vi "Write OVP_Enable.vi"(8 "error in":errorcluster, 10 "OVP_Enable":bool, 11 "36234A in":refnum<class "36234A.lvclass">) -> (0 "error out":errorcluster, 3 "36234A out":refnum<class "36234A.lvclass">)   [LabVIEW 2019, in "36234A.lvlib" / "36234A.lvclass"]
uses:
  Library/36234A.lvclass
  C:/Users/Public/Documents/Development/builds/Instruments/PowerSupply.lvlibp/Library/PowerSupply.lvclass
  builds/Instruments/PowerSupply.lvlibp/Accessors/Read Active Channel.vi
  builds/Instruments/PowerSupply.lvlibp/Library/PowerSupply.lvclass
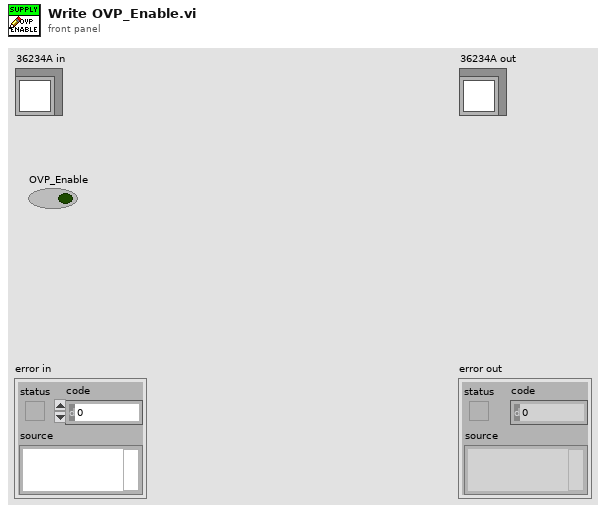
[diagram p1: front panel]
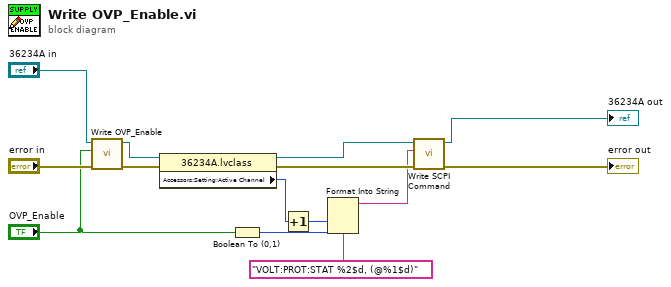
[diagram p0: block diagram]
diagram:
  n1 = call-parent "Write OVP_Enable.vi"("error in"="error in", "OVP_Enable"="OVP_Enable", "PowerSupply in"="36234A in") -> ("error out"=w14:errorcluster, "PowerSupply out"=w11:refnum<class "36234A.lvclass">)  [unwired: 7 in]
  n2 = property class="36234A.lvclass"(reference=w11, error in=w14) -> (reference out=w6:refnum<class "36234A.lvclass">, error out=w5:errorcluster, "Accessors:Setting:Active Channel"=w7:u32)
  n3 = Boolean To (0,1)(Boolean="OVP_Enable") -> (0, 1=w8:i16)
  n4 = Increment(x=w7) -> (x+1=w1:u32)
  n5 = Format Into String(format string="VOLT:PROT:STAT %2$d, (@%1$d)", w1, w8) -> (resulting string=w2:string)  [unwired: 2 in, 1 out]
  n6 = call "Write SCPI Command.vi"("error in (no error)"=w5, "SCPI Command"=w2, "36234A in"=w6) -> ("error out"=→"error out":errorcluster, "36234A out"=→"36234A out":refnum<class "36234A.lvclass">)  [unwired: 7 in]
